vi "Service.Create.vi"(7 "Type":T1, 8 "error in (no error)":errorcluster, 10 "Variant":variant, 11 "Section Ptr":T2 format="%.0x") -> (0 "error out":errorcluster, 3 "Parent Ref out":T2 format="%.0x")   [LabVIEW 2019, in "Diagnostics Addon System Explorer.lvlib"]
uses:
  Diagnostics Addon System Explorer.lvlib
  Shared/SubVIs/Constants.vi
  Shared/Diagnostics Addon Shared.lvlib
  <vilib>/NI/NI VeriStand Advanced SysDef API/SysDef API/Advanced System Definition.lvlib
  Types/FG.Action.ctl
  <vilib>/NI VeriStand/Custom Device API/Custom Device Channel Type.ctl
  <vilib>/NI VeriStand/Custom Device API/Custom Device API.lvlib
  <vilib>/NI VeriStand/Custom Device API/Custom Device Channel.ctl
  Shared/Types/DTC.Descriptor.ctl
  Shared/Types/DTC.Settings.ctl
  Shared/Types/Signal.ctl
  Types/Frame.Export.ctl
  Types/CmdResp.Export.ctl
  Types/IO.Export.ctl
  <vilib>/NI VeriStand/Custom Device API/Custom Device Item Ref.ctl
  Shared/Types/Type.ctl
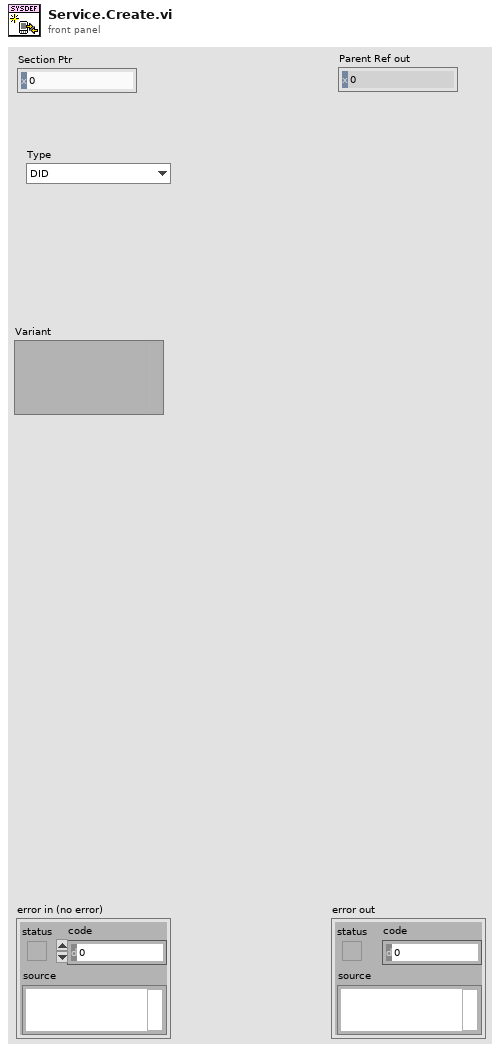
[diagram p1: front panel]
types:
  T1 = typedef "Diagnostics Addon Shared.lvlib/Type.ctl" = enum16{"DID", "CDID", "PID", "CPID", "Read Memory", "Write Memory", "IO Control", "Routine Start", "Routine Request", "Routine Stop", "User Defined", "DTC Control", "Clear DTCs", "Read DTCs", "Start DTCs", "DTC Change Count", "Tester Present", "Unlock ECU", "Reset ECU", "Diagnostic Session Control", "Normal Communication Control", "Configure and Start DPIDs", "Stop DPIDs"}
  T2 = typedef "Custom Device API.lvlib/Custom Device Item Ref.ctl" = u64
  T3 = typedef "Diagnostics Addon System Explorer.lvlib/Frame.Export.ctl" = cluster{"Name":string, "Description":string, "ID":u32, "Signals":T4[]}
  T4 = typedef "Diagnostics Addon Shared.lvlib/Signal.ctl" = cluster{"Start Bit":u32, "Length":u32, "Scaling Factor":dbl, "Scaling Offset":dbl, "Minimum":dbl, "Maximum":dbl, "Data Type":u32, "Byte Order":u32, "Default Value":dbl, "Name":string, "Units":string, "Description":string}
  T5 = typedef "Diagnostics Addon System Explorer.lvlib/FG.Action.ctl" = enum16{"Get", "Set"}
  T6 = typedef "Diagnostics Addon System Explorer.lvlib/IO.Export.ctl" = cluster{"Name":string, "Description":string, "ID":u16, "Signals":T7}
  T7 = typedef "Diagnostics Addon System Explorer.lvlib/CmdResp.Export.ctl" = cluster{"Cmd":T4[], "Response":T4[]}
  T8 = typedef "Diagnostics Addon Shared.lvlib/DTC.Settings.ctl" = cluster{"Descriptor":T9, "Value.Code":dbl[], "Value.String":string[], "Value.J2012String":string[], "Status.Code":dbl[], "Status.String":string[]}
  T9 = typedef "Diagnostics Addon Shared.lvlib/DTC.Descriptor.ctl" = cluster{"DTC Byte Length":i32, "Status Byte Length":i32, "Add Data Byte Length":i32, "Byte Order":enum16{"Motorola", "Intel"}}
  T10 = typedef "Custom Device API.lvlib/Custom Device Channel.ctl" = cluster{"Type":T11, "Units":string, "Default Value":dbl, "Faultable":bool, "Scalable":bool}
  T11 = typedef "Custom Device API.lvlib/Custom Device Channel Type.ctl" = enum16{"Input", "Output"}
  T12 = typedef "Diagnostics Addon Shared.lvlib/Protocol.ctl" = enum16{"GMLAN", "KWP-2000", "UDS", "User-Defined"}
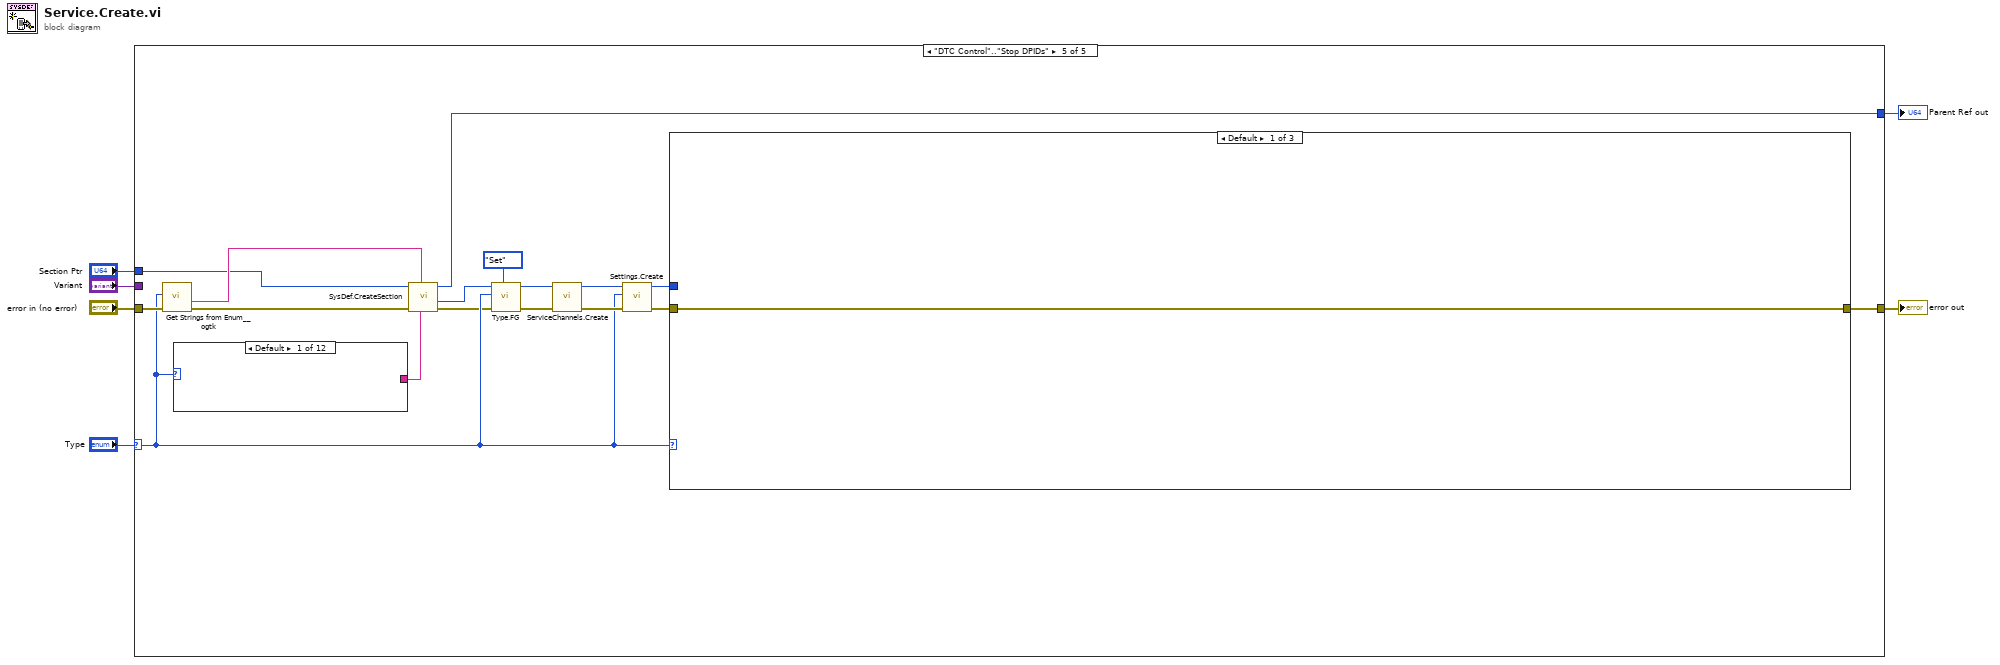
[diagram p0: block diagram]
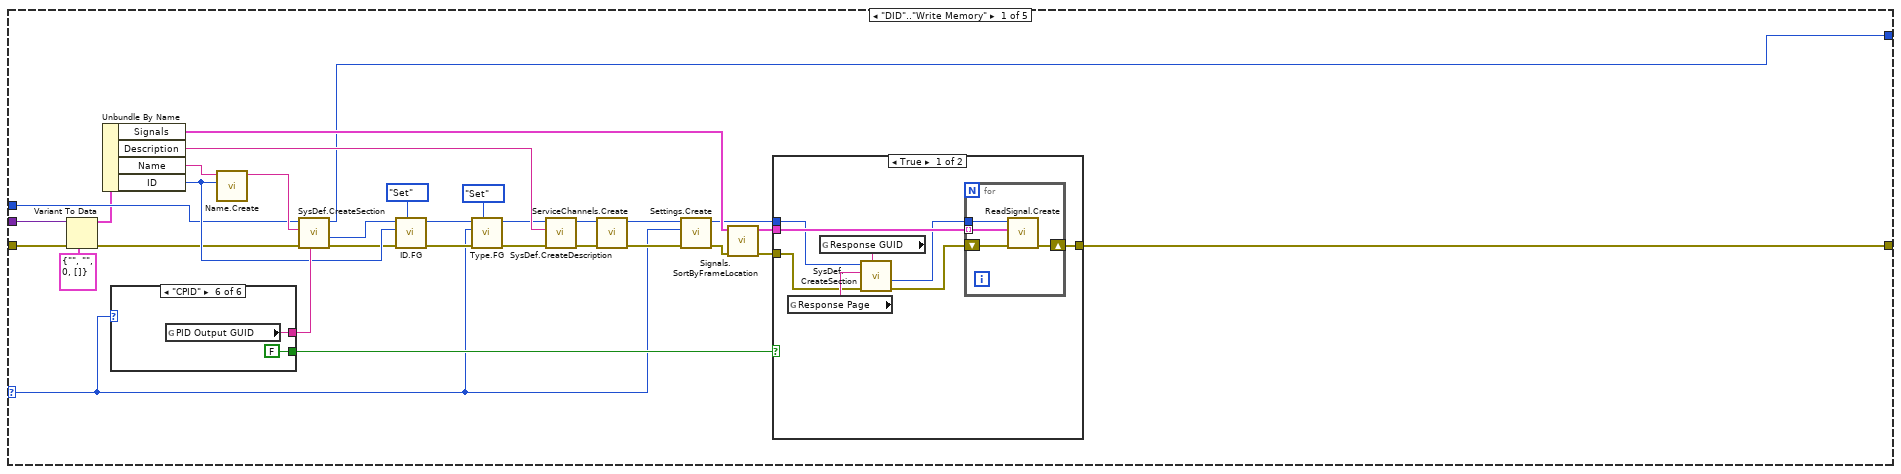
[diagram p2: hidden frame]
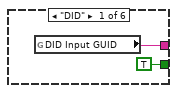
[diagram p3: hidden frame]
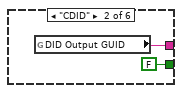
[diagram p4: hidden frame]
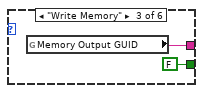
[diagram p5: hidden frame]
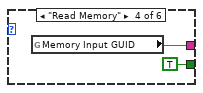
[diagram p6: hidden frame]
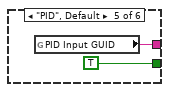
[diagram p7: hidden frame]
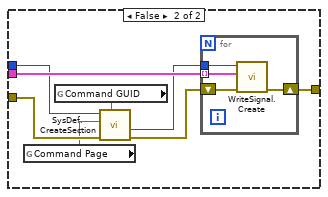
[diagram p8: hidden frame]
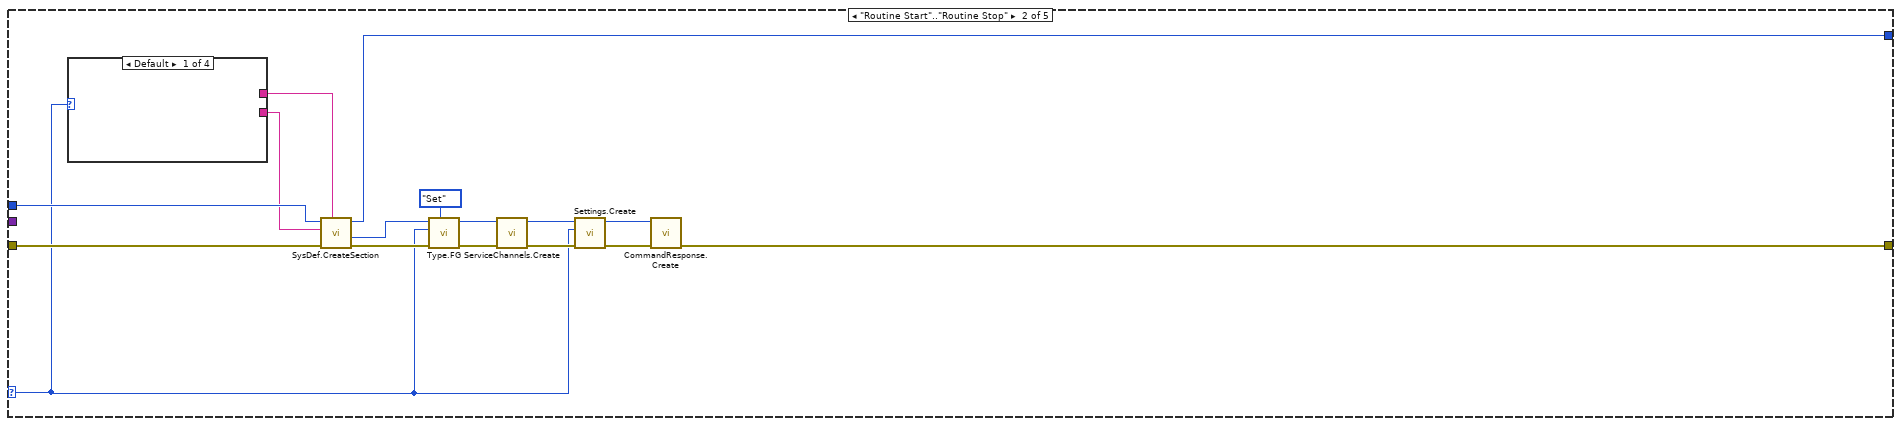
[diagram p9: hidden frame]
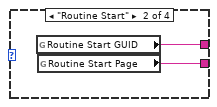
[diagram p10: hidden frame]
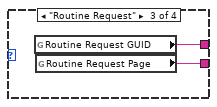
[diagram p11: hidden frame]
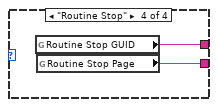
[diagram p12: hidden frame]
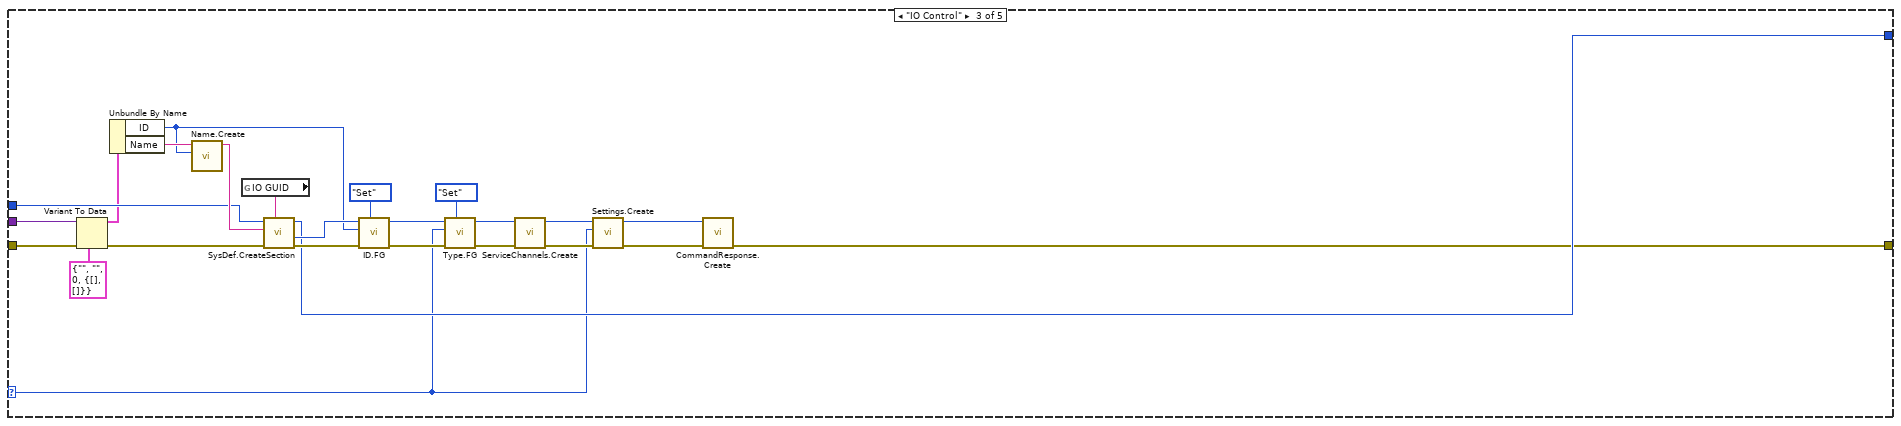
[diagram p13: hidden frame]
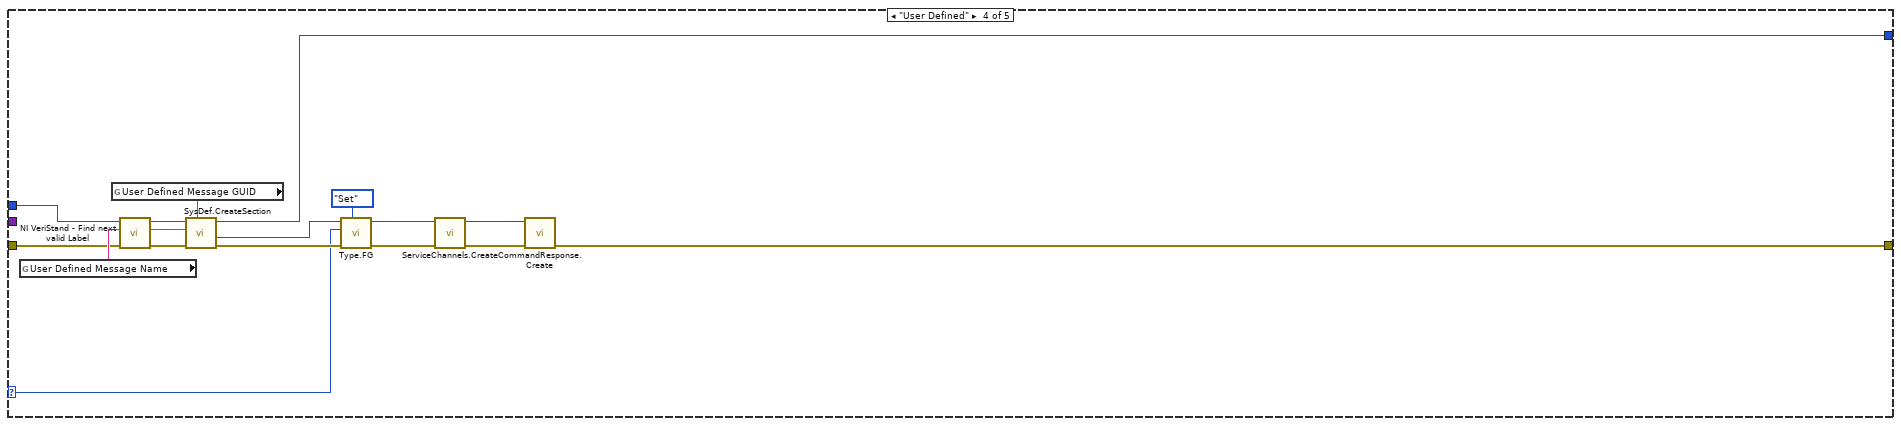
[diagram p14: hidden frame]
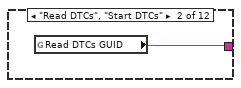
[diagram p15: hidden frame]
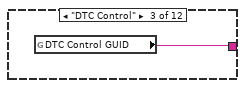
[diagram p16: hidden frame]
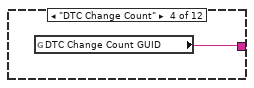
[diagram p17: hidden frame]
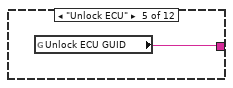
[diagram p18: hidden frame]
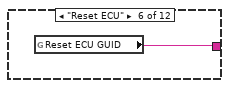
[diagram p19: hidden frame]
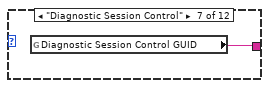
[diagram p20: hidden frame]
diagram:
  n1 = case shown="\"DTC Control\"..\"Stop DPIDs\"" "Type" {
    selector: "Type" -> [w13 w75 w99 w122 w147]
    tunnel: "error in (no error)" -> [w15 w90 w110 w133 w150]
    tunnel: "Section Ptr" -> [w14 w88 w114 w132 w143]
    tunnel: [w12 w89 w112 w131 w146] -> w3
    tunnel: [w11 w85 w113 w130 w145] -> w2
    tunnel: "Variant" -> [w9 _ w109 _ _]
    frame "DID".."Write Memory" {
      n2 = Variant To Data(error in=w15, type=T3 {"Name"="", "Description"="", "ID"=0, "Signals"=[]} ("Frame"), Variant=w9) -> (data=w7:T3, error out=w10:errorcluster)
      n3 = Unbundle By Name(w7) -> ("Signals"=w23:T4[], "Description"=w36:string, "Name"=w32:string, "ID"=w34:u32)
      n4 = case shown="\"CPID\"" w13 {
        tunnel: [w40 w42 w44 w46 w48 w50] -> w37
        tunnel: [TRUE FALSE FALSE TRUE TRUE FALSE] -> w31
        frame "DID" {
          n5 = global read "Constants.vi" "DID Input GUID"() -> (w40:string)
        }
        frame "CDID" {
          n6 = global read "Constants.vi" "DID Output GUID"() -> (w42:string)
        }
        frame "Write Memory" {
          n7 = global read "Constants.vi" "Memory Output GUID"() -> (w44:string)
        }
        frame "Read Memory" {
          n8 = global read "Constants.vi" "Memory Input GUID"() -> (w46:string)
        }
        frame "PID", Default {
          n9 = global read "Constants.vi" "PID Input GUID"() -> (w48:string)
        }
        frame "CPID" {
          n10 = global read "Constants.vi" "PID Output GUID"() -> (w50:string)
        }
      }
      n11 = call "Name.Create.vi"("PID Number"=w34, "PID Name"=w32) -> ("VS Name"=w38:string)  [unwired: 9 in]
      n12 = call <vilib>:"SysDef.CreateSection.vi"("GUID"=w37, "error in (no error)"=w10, "Name"=w38, "nodeID"=w14) -> ("error out"=w29:errorcluster, "New NodeID"=w30:u64, "nodeID out"=w11:u64)  [unwired: 4 in, 1 out]
      n13 = call "ID.FG.vi"("Action"=FG.Action."Set", "error in (no error)"=w29, "ID"=w34, "Device Item Ref in"=w30) -> ("error out"=w28:errorcluster, "Device Item Ref out"=w27:T2)  [unwired: 5 in, 1 out]
      n14 = call "Type.FG.vi"("Action"=FG.Action."Set", "error in (no error)"=w28, "Type"=w13, "Device Item Ref in"=w27) -> ("error out"=w25:errorcluster, "Device Item Ref out"=w26:T2)  [unwired: 5 in, 1 out]
      n15 = call <vilib>:"SysDef.CreateDescription.vi"("error in (no error)"=w25, "Description"=w36, "ID in"=w26) -> ("error out"=w21:errorcluster, "ID out"=w20:T2)  [unwired: 7 in]
      n16 = call "ServiceChannels.Create.vi"("error in (no error)"=w21, "nodeID in"=w20) -> ("error out"=w16:errorcluster, "nodeID out"=w18:u64)  [unwired: 8 in]
      n17 = call "Settings.Create.vi"("error in (no error)"=w16, "Type"=w13, "nodeID in"=w18) -> ("error out"=w17:errorcluster, "nodeID out"=w19:u64)  [unwired: 7 in]
      n18 = call "Signals.SortByFrameLocation.vi"("error in (no error)"=w17, "Signals in"=w23) -> ("error out"=w24:errorcluster, "Signals out"=w22:T4[])  [unwired: 8 in]
      n19 = case shown="True" w31 {
        tunnel: w19 -> [w51 w67]
        tunnel: w22 -> [w58 w70]
        tunnel: [w57 w69] -> w12
        tunnel: w24 -> [w53 w68]
        frame True {
          n20 = global read "Constants.vi" "Response Page"() -> (w55:string)
          n21 = global read "Constants.vi" "Response GUID"() -> (w56:string)
          n22 = call <vilib>:"SysDef.CreateSection.vi"("GUID"=w56, "error in (no error)"=w53, "Name"=w55, "nodeID"=w51) -> ("error out"=w54:errorcluster, "New NodeID"=w52:u64)  [unwired: 4 in, 2 out]
          n23 = for {
            shift-right: [w61] -> w57
            shift-left: w54 -> [w62]
            tunnel: w58 -> [w59] mode=indexing
            tunnel: w52 -> [w60]
            n24 = call "ReadSignal.Create.vi"("error in (no error)"=w62, "Signal Parameters"=w59, "Section Ptr"=w60) -> ("error out"=w61:errorcluster)  [unwired: 7 in, 1 out]
          }
        }
        frame False {
          n25 = global read "Constants.vi" "Command Page"() -> (w63:string)
          n26 = global read "Constants.vi" "Command GUID"() -> (w64:string)
          n27 = call <vilib>:"SysDef.CreateSection.vi"("GUID"=w64, "error in (no error)"=w68, "Name"=w63, "nodeID"=w67) -> ("error out"=w65:errorcluster, "New NodeID"=w66:u64)  [unwired: 4 in, 2 out]
          n28 = for {
            shift-right: [w71] -> w69
            shift-left: w65 -> [w73]
            tunnel: w70 -> [w72] mode=indexing
            tunnel: w66 -> [w74]
            n29 = call "WriteSignal.Create.vi"("error in (no error)"=w73, "Signal Parameters"=w72, "Section Ptr"=w74) -> ("error out"=w71:errorcluster)  [unwired: 7 in, 1 out]
          }
        }
      }
    }
    frame "Routine Start".."Routine Stop" {
      n30 = case shown="Default" w75 {
        tunnel: [_ w92 w94 w96] -> w87
        tunnel: [_ w91 w93 w95] -> w86
        frame Default {
        }
        frame "Routine Start" {
          n31 = global read "Constants.vi" "Routine Start GUID"() -> (w92:string)
          n32 = global read "Constants.vi" "Routine Start Page"() -> (w91:string)
        }
        frame "Routine Request" {
          n33 = global read "Constants.vi" "Routine Request GUID"() -> (w94:string)
          n34 = global read "Constants.vi" "Routine Request Page"() -> (w93:string)
        }
        frame "Routine Stop" {
          n35 = global read "Constants.vi" "Routine Stop GUID"() -> (w96:string)
          n36 = global read "Constants.vi" "Routine Stop Page"() -> (w95:string)
        }
      }
      n37 = call <vilib>:"SysDef.CreateSection.vi"("GUID"=w87, "error in (no error)"=w90, "Name"=w86, "nodeID"=w88) -> ("error out"=w78:errorcluster, "New NodeID"=w79:u64, "nodeID out"=w85:u64)  [unwired: 4 in, 1 out]
      n38 = call "Type.FG.vi"("Action"=FG.Action."Set", "error in (no error)"=w78, "Type"=w75, "Device Item Ref in"=w79) -> ("error out"=w77:errorcluster, "Device Item Ref out"=w76:T2)  [unwired: 5 in, 1 out]
      n39 = call "ServiceChannels.Create.vi"("error in (no error)"=w77, "nodeID in"=w76) -> ("error out"=w84:errorcluster, "nodeID out"=w83:u64)  [unwired: 8 in]
      n40 = call "Settings.Create.vi"("error in (no error)"=w84, "Type"=w75, "nodeID in"=w83) -> ("error out"=w81:errorcluster, "nodeID out"=w80:u64)  [unwired: 7 in]
      n41 = call "CommandResponse.Create.vi"("error in (no error)"=w81, "New NodeID"=w80) -> ("error out"=w89:errorcluster)  [unwired: 9 in]
    }
    frame "IO Control" {
      n42 = Variant To Data(error in=w110, type=T6 {"Name"="", "Description"="", "ID"=0, "Signals"={"Cmd"=[], "Response"=[]}} ("IO Control"), Variant=w109) -> (data=w108:T6, error out=w111:errorcluster)
      n43 = Unbundle By Name(w108) -> ("ID"=w116:u16, "Name"=w119:string)
      n44 = call "Name.Create.vi"("PID Number"=w116, "PID Name"=w119) -> ("VS Name"=w121:string)  [unwired: 9 in]
      n45 = global read "Constants.vi" "IO GUID"() -> (w120:string)
      n46 = call <vilib>:"SysDef.CreateSection.vi"("GUID"=w120, "error in (no error)"=w111, "Name"=w121, "nodeID"=w114) -> ("error out"=w118:errorcluster, "New NodeID"=w117:u64, "nodeID out"=w113:u64)  [unwired: 4 in, 1 out]
      n47 = call "ID.FG.vi"("Action"=FG.Action."Set", "error in (no error)"=w118, "ID"=w116, "Device Item Ref in"=w117) -> ("error out"=w101:errorcluster, "Device Item Ref out"=w98:T2)  [unwired: 5 in, 1 out]
      n48 = call "Type.FG.vi"("Action"=FG.Action."Set", "error in (no error)"=w101, "Type"=w99, "Device Item Ref in"=w98) -> ("error out"=w100:errorcluster, "Device Item Ref out"=w97:T2)  [unwired: 5 in, 1 out]
      n49 = call "ServiceChannels.Create.vi"("error in (no error)"=w100, "nodeID in"=w97) -> ("error out"=w106:errorcluster, "nodeID out"=w105:u64)  [unwired: 8 in]
      n50 = call "Settings.Create.vi"("error in (no error)"=w106, "Type"=w99, "nodeID in"=w105) -> ("error out"=w103:errorcluster, "nodeID out"=w104:u64)  [unwired: 7 in]
      n51 = call "CommandResponse.Create.vi"("error in (no error)"=w103, "New NodeID"=w104) -> ("error out"=w112:errorcluster)  [unwired: 9 in]
    }
    frame "User Defined" {
      n52 = global read "Constants.vi" "User Defined Message Name"() -> (w136:string)
      n53 = global read "Constants.vi" "User Defined Message GUID"() -> (w138:string)
      n54 = call <vilib>:"NI VeriStand - Find next valid Label.vi"("error in (no error)"=w133, "Label"=w136, "Item Ref in"=w132) -> ("error out"=w135:errorcluster, "Label out"=w134:string, "Item Ref out"=w137:T2)  [unwired: 4 in, 2 out]
      n55 = call <vilib>:"SysDef.CreateSection.vi"("GUID"=w138, "error in (no error)"=w135, "Name"=w134, "nodeID"=w137) -> ("error out"=w123:errorcluster, "New NodeID"=w124:u64, "nodeID out"=w130:u64)  [unwired: 4 in, 1 out]
      n56 = call "Type.FG.vi"("Action"=FG.Action."Set", "error in (no error)"=w123, "Type"=w122, "Device Item Ref in"=w124) -> ("error out"=w126:errorcluster, "Device Item Ref out"=w125:T2)  [unwired: 5 in, 1 out]
      n57 = call "ServiceChannels.Create.vi"("error in (no error)"=w126, "nodeID in"=w125) -> ("error out"=w129:errorcluster, "nodeID out"=w128:u64)  [unwired: 8 in]
      n58 = call "CommandResponse.Create.vi"("error in (no error)"=w129, "New NodeID"=w128) -> ("error out"=w131:errorcluster)  [unwired: 9 in]
    }
    frame "DTC Control".."Stop DPIDs" {
      n59 = call <userlib>:"Get Strings from Enum__ogtk.vi"("error in (no error)"=w150, "Enum"=w147) -> ("error out"=w144:errorcluster, "String Value"=w149:string)  [unwired: 6 in, 2 out]
      n60 = case shown="Default" w147 {
        tunnel: [_ w156 w157 w158 w159 w160 w161 w162 w163 w164 w165 w166] -> w151
        frame Default {
        }
        frame "Read DTCs", "Start DTCs" {
          n61 = global read "Constants.vi" "Read DTCs GUID"() -> (w156:string)
        }
        frame "DTC Control" {
          n62 = global read "Constants.vi" "DTC Control GUID"() -> (w157:string)
        }
        frame "DTC Change Count" {
          n63 = global read "Constants.vi" "DTC Change Count GUID"() -> (w158:string)
        }
        frame "Unlock ECU" {
          n64 = global read "Constants.vi" "Unlock ECU GUID"() -> (w159:string)
        }
        frame "Reset ECU" {
          n65 = global read "Constants.vi" "Reset ECU GUID"() -> (w160:string)
        }
        frame "Diagnostic Session Control" {
          n66 = global read "Constants.vi" "Diagnostic Session Control GUID"() -> (w161:string)
        }
        frame "Normal Communication Control" {
          n67 = global read "Constants.vi" "Normal Communication Control GUID"() -> (w162:string)
        }
        frame "Configure and Start DPIDs" {
          n68 = global read "Constants.vi" "Configure and Start DPIDs GUID"() -> (w163:string)
        }
        frame "Stop DPIDs" {
          n69 = global read "Constants.vi" "Stop DPIDs GUID"() -> (w164:string)
        }
        frame "Clear DTCs" {
          n70 = global read "Constants.vi" "Clear DTCs GUID"() -> (w165:string)
        }
        frame "Tester Present" {
          n71 = global read "Constants.vi" "Tester Present GUID"() -> (w166:string)
        }
      }
      n72 = call <vilib>:"SysDef.CreateSection.vi"("GUID"=w151, "error in (no error)"=w144, "Name"=w149, "nodeID"=w143) -> ("error out"=w142:errorcluster, "New NodeID"=w141:u64, "nodeID out"=w145:u64)  [unwired: 4 in, 1 out]
      n73 = call "Type.FG.vi"("Action"=FG.Action."Set", "error in (no error)"=w142, "Type"=w147, "Device Item Ref in"=w141) -> ("error out"=w140:errorcluster, "Device Item Ref out"=w139:T2)  [unwired: 5 in, 1 out]
      n74 = call "ServiceChannels.Create.vi"("error in (no error)"=w140, "nodeID in"=w139) -> ("error out"=w154:errorcluster, "nodeID out"=w155:u64)  [unwired: 8 in]
      n75 = call "Settings.Create.vi"("error in (no error)"=w154, "Type"=w147, "nodeID in"=w155) -> ("error out"=w153:errorcluster, "nodeID out"=w152:u64)  [unwired: 7 in]
      n76 = case shown="Default" w147 {
        tunnel: [w167 w169 w190] -> w146
        tunnel: w152 -> [_ w170 w188]
        tunnel: w153 -> [w167 w168 w189]
        frame Default {
        }
        frame "DTC Control" {
          n77 = global read "Constants.vi" "Command Page"() -> (w172:string)
          n78 = global read "Constants.vi" "Command GUID"() -> (w171:string)
          n79 = call <vilib>:"SysDef.CreateSection.vi"("GUID"=w171, "error in (no error)"=w168, "Name"=w172, "nodeID"=w170) -> ("error out"=w169:errorcluster)  [unwired: 4 in, 3 out]
        }
        frame "Read DTCs", "Start DTCs" {
          n80 = call "CAN.Protocol.Find.vi"("error in (no error)"=w189, "Node Ptr"=w188) -> ("error out"=w182:errorcluster, "Diagnostic Protocol"=w187:T12, "Section Ref out"=w183:T2)  [unwired: 7 in]
          n81 = case shown="\"User-Defined\"" w187 {
            tunnel: [u32 2 ("Mode ID") u32 3 ("Mode ID") w198 u32 2 ("Mode ID")] -> w181
            tunnel: [u32 1 ("Mode ID") u32 1 ("Mode ID") w198 u32 1 ("Mode ID")] -> w180
            tunnel: [u32 0 ("Mode ID") u32 0 ("Mode ID") w198 u32 0 ("Mode ID")] -> w179
            frame "GMLAN" {
            }
            frame "UDS" {
            }
            frame "User-Defined" {
              w198 = u8 0 ("Mode ID")
            }
            frame "KWP-2000" {
            }
          }
          n82 = Bundle By Name(cluster=T8 {"Descriptor"={"DTC Byte Length"=2, "Status Byte Length"=1, "Add Data Byte Length"=1, "Byte Order"=enum."Motorola"}, "Value.Code"=[], "Value.String"=[], "Value.J2012String"=[], "Status.Code"=[], "Status.String"=[]} ("DTC"), "Descriptor.DTC Byte Length"=w181, "Descriptor.Status Byte Length"=w180, "Descriptor.Add Data Byte Length"=w179) -> (w184:T8)
          n83 = call "DTCDescriptor.FG.vi"("Action"=FG.Action."Set", "error in (no error)"=w182, "DTC"=w184, "Device Item Ref in"=w183) -> ("error out"=w177:errorcluster, "Device Item Ref out"=w176:T2)  [unwired: 5 in, 1 out]
          n84 = global read "Constants.vi" "Response Page"() -> (w173:string)
          n85 = global read "Constants.vi" "Response GUID"() -> (w178:string)
          n86 = call <vilib>:"SysDef.CreateSection.vi"("GUID"=w178, "error in (no error)"=w177, "Name"=w173, "nodeID"=w176) -> ("error out"=w175:errorcluster, "New NodeID"=w174:u64)  [unwired: 4 in, 2 out]
          n87 = for {
            N: u32 10 ("t") -> [_]
            tunnel: w174 -> [w214]
            shift-right: [w218] -> w190
            shift-left: w175 -> [w213]
            i -> [w217]
            n88 = global read "Constants.vi" "DTC_Signal Suffix"() -> (w211:string[])
            n89 = global read "Constants.vi" "DTC_Signal Prefix"() -> (w210:string)
            n90 = Increment(x=w217) -> (x+1=w216:i32)
            n91 = Number To Decimal String(number=w216) -> (decimal integer string=w215:string)  [unwired: 1 in]
            n92 = Concatenate Strings(w210, w215) -> (w212:string)
            n93 = global read "Constants.vi" "DTC GUID"() -> (w209:string)
            n94 = call <vilib>:"SysDef.CreateSection.vi"("GUID"=w209, "error in (no error)"=w213, "Name"=w212, "nodeID"=w214) -> ("error out"=w204:errorcluster, "New NodeID"=w202:u64)  [unwired: 4 in, 2 out]
            n95 = global read "Constants.vi" "DTCs_# of DTCs"() -> (w207:string)
            n96 = global read "Constants.vi" "Protected Signal GUID"() -> (w206:string)
            n97 = call <vilib>:"SysDef.CreateChannel.vi"("GUID"=w206, "error in (no error)"=w204, "Channel"=T10 {"Type"=enum."Output", "Units"="", "Default Value"=0.0, "Faultable"=FALSE, "Scalable"=FALSE}, "Name"=w207, "nodeID"=w202) -> ("error out"=w205:errorcluster, "nodeID out"=w203:u64)  [unwired: 3 in, 2 out]
            n98 = for {
              tunnel: w203 -> [w224]
              tunnel: w212 -> [w221]
              tunnel: w211 -> [w222] mode=indexing
              shift-right: [w226] -> w218
              shift-left: w205 -> [w223]
              n99 = global read "Constants.vi" "Protected Signal GUID"() -> (w219:string)
              n100 = Concatenate Strings(w221, w222) -> (w220:string)
              n101 = call <vilib>:"SysDef.CreateChannel.vi"("GUID"=w219, "error in (no error)"=w223, "Channel"=T10 {"Type"=enum."Output", "Units"="", "Default Value"=0.0, "Faultable"=FALSE, "Scalable"=FALSE}, "Name"=w220, "nodeID"=w224) -> ("error out"=w226:errorcluster)  [unwired: 3 in, 3 out]
            }
          }
        }
      }
    }
  }
  "error out" <- w3
  "Parent Ref out" <- w2
